vi "Update Service.vi"(8 "error in (no error)":errorcluster, 9 "data":string, 10 "Service Name":string, 11 "DIMActor in":refnum<class "DIMActor.lvclass">) -> (0 "error out":errorcluster, 3 "DIMActor out":refnum<class "DIMActor.lvclass">)   [LabVIEW 2012, in "DIMActor.lvlib" / "DIMActor.lvclass"]
uses:
  DIMActor.lvclass
  DIMActor.lvclass/DIMActor.ctl
  SVN/LV2009/GPL/lib.lib/DimLVEvent/LVDimInterface/LVDimInterface.lvlib
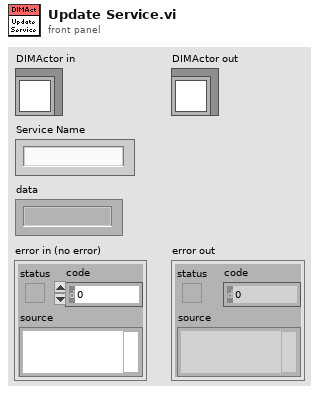
[diagram p1: front panel]
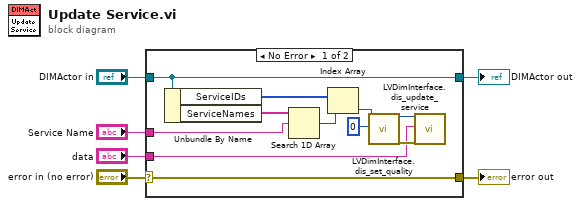
[diagram p0: block diagram]
diagram:
  n1 = case shown="No Error" "error in (no error)" {
    selector: "error in (no error)" -> [w17 w19]
    tunnel: [w17 w19] -> w5
    tunnel: [w13 w18] -> w3
    tunnel: "DIMActor in" -> [w13 w18]
    tunnel: "Service Name" -> [w11 _]
    tunnel: "data" -> [w7 _]
    frame No Error {
      n2 = Unbundle By Name(w13) -> ("ServiceIDs"=w10:i32[], "ServiceNames"=w12:string[])
      n3 = Search 1D Array(1D array=w12, element=w11) -> (index of element=w9:i32)  [unwired: 1 in]
      n4 = Index Array(array=w10, index=w9) -> (element=w8:i32)
      n5 = call "LVDimInterface.dis_set_quality.vi"("my_serviceID"=w8, "quality"=0) -> ("my_serviceID (out)"=w14:i32, "error out"=w16:errorcluster)  [unwired: 16 in]
      n6 = call "LVDimInterface.dis_update_service.vi"("my_serviceID"=w14, "data"=w7, "error in (no error)"=w16) -> ()  [unwired: 14 in, 3 out]
    }
    frame Error {
    }
  }
  "error out" <- w5
  "DIMActor out" <- w3
